vi "Determine Warnings 3-5.vi"() -> ()   [LabVIEW 2014]
panel:
  out "Warning?":bool
  out "Warning Text":string
  in  "Min Temp":dbl
  in  "Max Temp":dbl
  in  "Current Temp":dbl
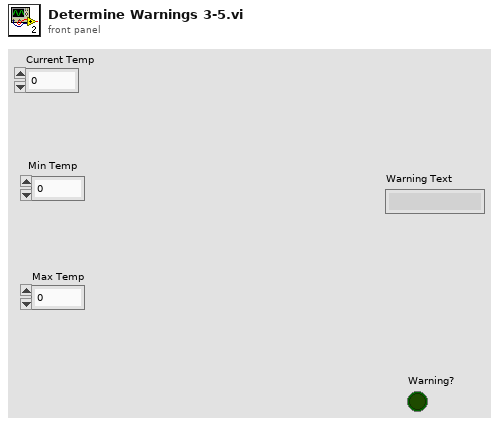
[diagram p1: front panel]
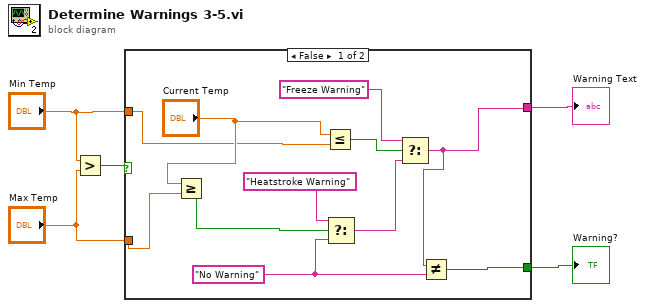
[diagram p0: block diagram]
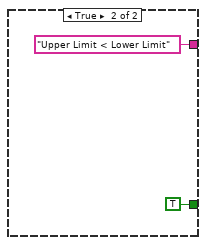
[diagram p2: hidden frame]
diagram:
  n1 = Greater?(x="Min Temp", y="Max Temp") -> (0:w3:bool)
  n2 = case shown="False" w3 {
    tunnel: "Min Temp" -> [w10 _]
    tunnel: "Max Temp" -> [w9 _]
    tunnel: [w8 TRUE] -> w2
    tunnel: [w7 "Upper Limit < Lower Limit" ("Warning Text")] -> w1
    frame False {
      w16 = "No Warning" ("Warning Text")
      n3 = Greater Or Equal?(x="Current Temp", y=w9) -> (x >= y?=w6:bool)
      n4 = Less Or Equal?(x="Current Temp", y=w10) -> (x <= y?=w12:bool)
      n5 = Select(t="Heatstroke Warning" ("Warning Text"), s=w6, f=w16) -> (s? t:f=w15:string)
      n6 = Select(t="Freeze Warning" ("Warning Text"), s=w12, f=w15) -> (s? t:f=w7:string)
      n7 = Not Equal?(x=w7, y=w16) -> (x != y?=w8:bool)
    }
    frame True {
    }
  }
  "Warning?" <- w2
  "Warning Text" <- w1
